vi "Export to Config.vi"(7 "selected path":path, 8 "error in":errorcluster, 11 "Device Ref in":T1 format="%.0x") -> (0 "error out":errorcluster)   [LabVIEW 2015, in "Modbus Master System Explorer.lvlib"]
uses:
  Modbus Master System Explorer.lvlib
  <vilib>/NI Veristand/Custom Device API/Custom Device Item Ref.ctl
  <vilib>/Utility/config.llb/NI_LVConfig.lvlib
  <vilib>/NI VeriStand/Custom Device API/Custom Device API.lvlib
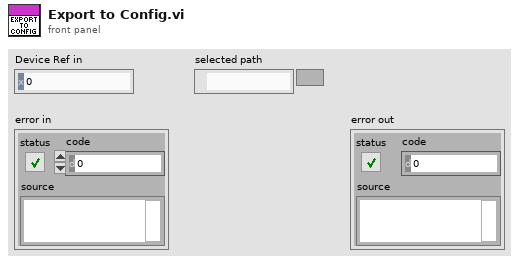
[diagram p1: front panel]
types:
  T1 = typedef "Custom Device API.lvlib/Custom Device Item Ref.ctl" = u64
  T2 = typedef "NI_LVConfig.lvlib/Config Data RefNum.ctl" = refnum<k1>
  T3 = typedef "Modbus Master Shared.lvlib/Channel Data.ctl" = cluster{"Coils":T4[], "Discrete Inputs":T4[], "Input Registers":T4[], "Holding Registers":T4[]}
  T4 = typedef "Modbus Master Shared.lvlib/Channel.ctl" = cluster{"Name":string, "Modbus Type":T5, "Veristand Type":T6, "Mapping":T7}
  T5 = typedef "Modbus Master Shared.lvlib/Modbus Type.ctl" = enum16{"Coil", "Discrete Input", "Holding Register", "Input Register"}
  T6 = typedef "Custom Device API.lvlib/Custom Device Channel Type.ctl" = enum16{"Input", "Output"}
  T7 = typedef "Modbus Master Shared.lvlib/Mapping.ctl" = cluster{"DataType":T8, "Starting Address":u16, "Sub-Index (Bool)":u16, "VS Reference":T1}
  T8 = typedef "Modbus Master Shared.lvlib/DataType.ctl" = enum16{"Double", "Single", "I64", "I32", "I16", "I8", "U64", "U32", "U16", "U8", "Boolean"}
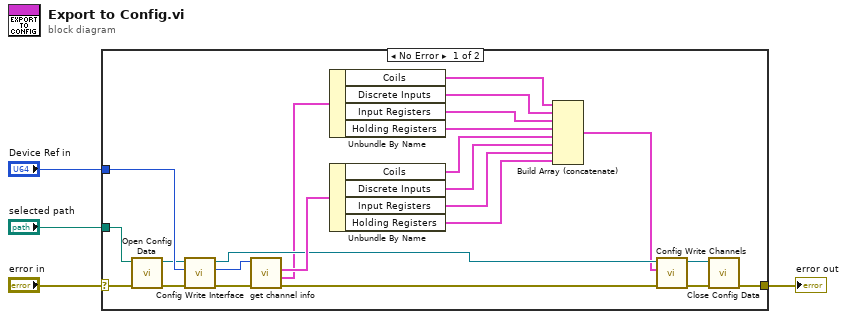
[diagram p0: block diagram]
diagram:
  n1 = case shown="No Error" "error in" {
    selector: "error in" -> [w16 w28]
    tunnel: "selected path" -> [w25 _]
    tunnel: [w20 w28] -> w3
    tunnel: "Device Ref in" -> [w26 _]
    frame No Error {
      n2 = call <vilib>:"Open Config Data.vi"("error in (no error)"=w16, "configuration file path"=w25) -> ("error out"=w15:errorcluster, "refnum"=w24:T2)  [unwired: 7 in, 1 out]
      n3 = call "Config Write Interface.vi"("error in (no error)"=w15, "Device Ref in"=w26, "Refnum in"=w24) -> ("error out"=w18:errorcluster, "Device Ref out"=w22:T1, "Refnum out"=w23:T2)  [unwired: 6 in]
      n4 = call "get channel info.vi"("error in (no error)"=w18, "Item Ref in"=w22) -> ("error out"=w17:errorcluster, "Outputs"=w14:T3, "Inputs"=w27:T3)  [unwired: 6 in, 1 out]
      n5 = Unbundle By Name(w14) -> ("Coils"=w13:T4[], "Discrete Inputs"=w12:T4[], "Input Registers"=w11:T4[], "Holding Registers"=w10:T4[])
      n6 = Unbundle By Name(w27) -> ("Coils"=w9:T4[], "Discrete Inputs"=w8:T4[], "Input Registers"=w7:T4[], "Holding Registers"=w6:T4[])
      n7 = Build Array (concatenate)(w13, w12, w11, w10, w9, w8, w7, w6) -> (w5:T4[])
      n8 = call "Config Write Channels.vi"("error in (no error)"=w17, "Channels In"=w5, "Refnum in"=w23) -> ("error out"=w21:errorcluster, "Refnum out"=w19:T2)  [unwired: 7 in]
      n9 = call <vilib>:"Close Config Data.vi"("error in (no error)"=w21, "refnum"=w19) -> ("error out"=w20:errorcluster)  [unwired: 8 in, 1 out]
    }
    frame Error {
    }
  }
  "error out" <- w3
